vi "Timed_Error_dialog.vi"(2 "Message":string, 3 "Seconds to wait":dbl=1.0 format="%.2f") -> (0 "Ignore":bool, 1 "Abort":bool)   [LabVIEW 2010]
doc: "Waits the number of seconds specified by the Seconds to Wait input, divided by the time dilation factor, if used."
panel:
  in  "Ignore Error":bool
  in  "Abort":bool
  out "Seconds waited":u32(slide) scale=0.0..30.0
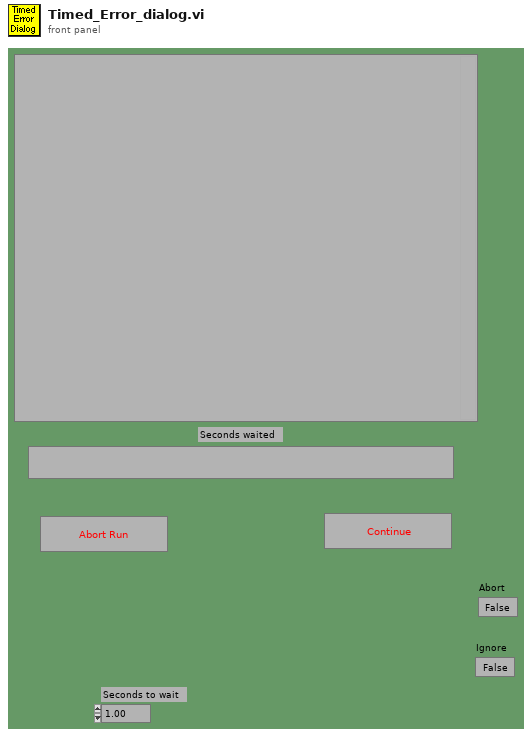
[diagram p1: front panel]
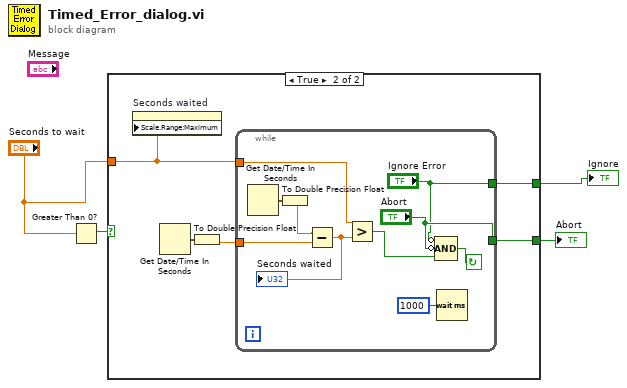
[diagram p0: block diagram]
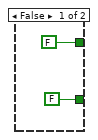
[diagram p2: hidden frame]
diagram:
  n1 = Greater Than 0?(x="Seconds to wait") -> (x > 0?=w3:bool)
  n2 = case shown="True" w3 {
    tunnel: [FALSE ("stop") w11] -> w4
    tunnel: "Seconds to wait" -> [_ w9]
    tunnel: [FALSE ("Ignore Error") w7] -> w1
    frame False {
    }
    frame True {
      n3 = property on="Seconds waited" class="Slide (strict)"("Scale.Range:Maximum"=w9) -> ()  [unwired: 2 in, 2 out]
      n4 = Get Date/Time In Seconds() -> (seconds since 1Jan1904=w8:timestamp)
      n5 = To Double Precision Float(number=w8) -> (double precision float=w10:dbl)
      n6 = while {
        tunnel: ["Abort"] -> w11
        tunnel: w9 -> [w17]
        tunnel: w10 -> [w21]
        tunnel: ["Ignore Error"] -> w7
        stop <- w19 continue-if-true
        n7 = Get Date/Time In Seconds() -> (seconds since 1Jan1904=w13:timestamp)
        n8 = To Double Precision Float(number=w13) -> (double precision float=w14:dbl)
        n9 = Subtract(x=w14, y=w21) -> (x-y=w16:dbl)
        "Seconds waited" <- w16
        n10 = Greater?(x=w17, y=w16) -> (0:w20:bool)
        n11 = Compound Arithmetic op=AND(invert "Ignore Error", invert "Abort", w20) -> (w19:bool)
        n12 = Wait (ms)(milliseconds to wait=u32 1000) -> ()  [unwired: 1 out]
      }
    }
  }
  "Abort" <- w4
  "Ignore" <- w1
